vi "Get All Paths in Variant.vi"(8 "error in (no error)":errorcluster, 11 "Variant in":variant) -> (0 "error out":errorcluster, 2 "Paths out":string[](array[string]), 3 "Variant out":variant)   [LabVIEW 2020, in "Variant Data Manipulation.lvlib"]
uses:
  Variant Data Manipulation.lvlib
  <vilib>/Utility/Data Type/NI_Data Type.lvlib
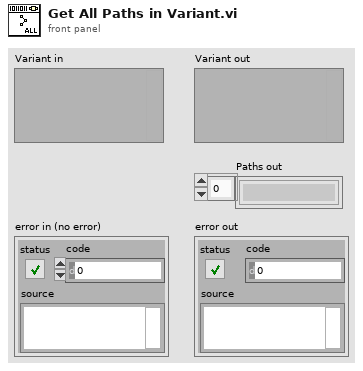
[diagram p1: front panel]
types:
  T1 = typedef "NI_Data Type.lvlib/Data Type.ctl" = enum8{"Invalid Type", "Void", "I8", "I16", "I32", "I64", "U8", "U16", "U32", "U64", "Single Float", "Double Float", "Extended Float", "Single Complex", "Double Complex", "Extended Complex", "Enum U8", "Enum U16", "Enum U32", "Enum U64", "Single Float With Unit", "Double Float With Unit", "Extended Float With Unit", "Single Complex with Unit", "Double Complex with Unit", "Extended Complex with Unit", "Boolean", "String", "Path", "Picture", "Tag", "Array", "Cluster", "Variant", "LV Variant", "Waveform", "Timestamp", "Digital Waveform", "Digital Data", "ExpressData", "Refnum", "External Data", "VI", "Poly VI", "LabVIEW Class Instance", "Fixed Point", "Set Collection", "Map Collection"}
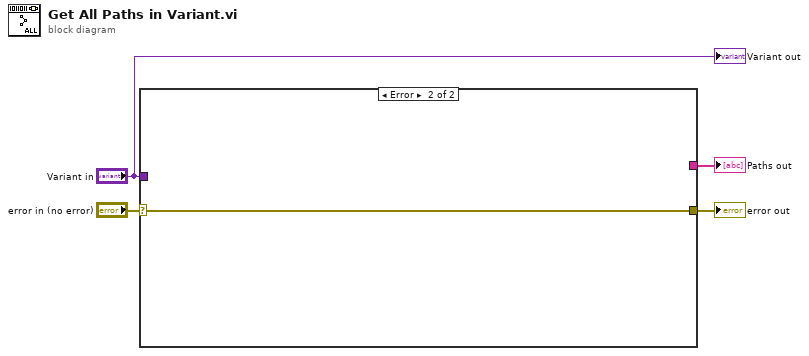
[diagram p0: block diagram]
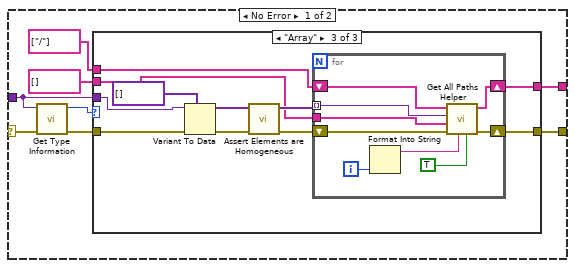
[diagram p2: hidden frame]
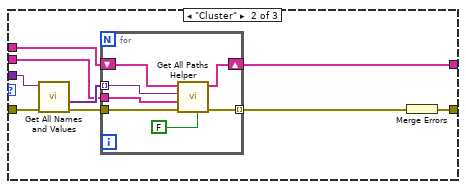
[diagram p4: hidden frame]
diagram:
  n1 = case shown="Error" "error in (no error)" {
    selector: "error in (no error)" -> [w6 w51]
    tunnel: [w12 _] -> w4
    tunnel: [w9 w51] -> w3
    tunnel: "Variant in" -> [w8 _]
    frame No Error {
      n2 = call <vilib>:"Get Type Information.vi"("error in (no error)"=w6, "variant"=w8) -> ("error out"=w5:errorcluster, "type"=w7:T1)  [unwired: 5 in, 3 out]
      n3 = case shown="\"Array\"" w7 {
        tunnel: w5 -> [w14 w16 w37]
        tunnel: [w14 w20 w41] -> w9
        tunnel: w8 -> [_ w23 w39]
        tunnel: string[] [] ("Array 3") -> [_ w19 w33]
        tunnel: string[] ["/"] ("Paths in") -> [w13 w18 w32]
        tunnel: [w13 w17 w31] -> w12
        frame Default {
        }
        frame "Cluster" {
          n4 = call "Get All Names and Values.vi"("error in"=w16, "Cluster in"=w23) -> ("error out"=w15:errorcluster, "Values"=w22:variant[])  [unwired: 5 in, 3 out]
          n5 = for {
            tunnel: w22 -> [w30] mode=indexing
            tunnel: [w29] -> w21 mode=indexing
            shift-right: [w24] -> w17
            shift-left: w18 -> [w25]
            tunnel: w15 -> [w27]
            tunnel: w19 -> [w26]
            n6 = call "Get All Paths Helper.vi"("is array element?"=FALSE ("first call?"), "error in (no error)"=w27, "parents"=w26, "Variant"=w30, "Paths in"=w25) -> ("error out"=w29:errorcluster, "Paths out"=w24:string[])  [unwired: 5 in]
          }
          n7 = Merge Errors(w21) -> (w20:errorcluster)
        }
        frame "Array" {
          n8 = Variant To Data(error in=w37, type=variant[] [], Variant=w39) -> (data=w38:variant[], error out=w36:errorcluster)
          n9 = call "Assert Elements are Homogeneous.vi"("error in (no error)"=w36, "array in"=w38) -> ("error out"=w34:errorcluster, "array out"=w35:variant[])  [unwired: 8 in]
          n10 = for {
            tunnel: w35 -> [w47] mode=indexing
            shift-right: [w50] -> w41
            shift-left: w34 -> [w49]
            shift-right: [w43] -> w31
            shift-left: w32 -> [w42]
            tunnel: w33 -> [w44]
            i -> [w46]
            n11 = Format Into String(w46) -> (resulting string=w45:string)  [unwired: 3 in, 1 out]
            n12 = call "Get All Paths Helper.vi"("is array element?"=TRUE ("first call?"), "index string"=w45, "error in (no error)"=w49, "parents"=w44, "Variant"=w47, "Paths in"=w42) -> ("error out"=w50:errorcluster, "Paths out"=w43:string[])  [unwired: 4 in]
          }
        }
      }
    }
    frame Error {
    }
  }
  "Paths out" <- w4
  "error out" <- w3
  "Variant out" <- "Variant in"
